vi "Add Item.vi"(0 "Monkeys in":T1, 1 "Item":u64, 2 "Monkey":string) -> (3 "Monkeys out":T1)   [LabVIEW 2020, in "AoC 2022.lvlib"]
uses:
  AoC 2022.lvlib
  Monkeys.ctl
  Monkey.ctl
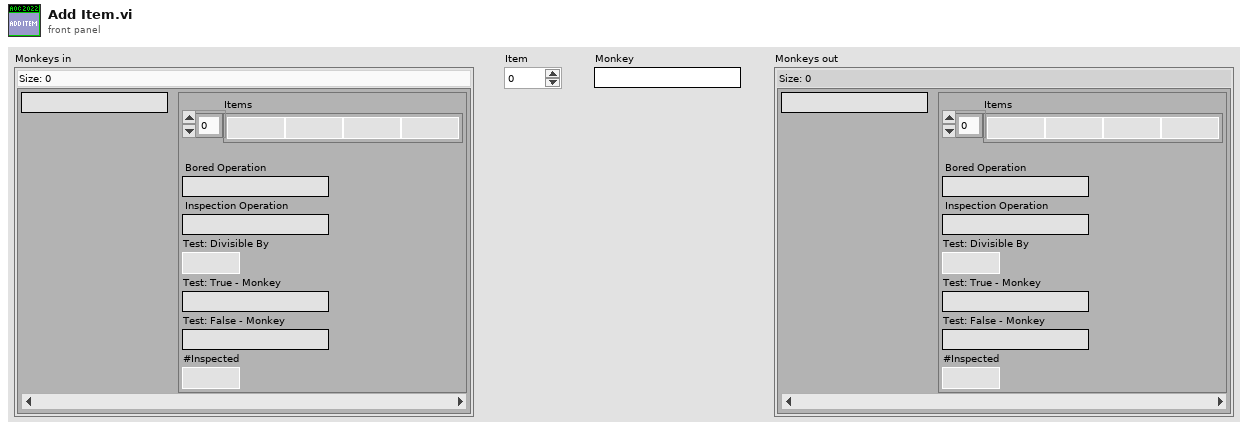
[diagram p1: front panel]
types:
  T1 = typedef "AoC 2022.lvlib/Monkeys.ctl" = map{string, T2}
  T2 = typedef "AoC 2022.lvlib/Monkey.ctl" = cluster{"Items":u64[], "Bored Operation":string, "Inspection Operation":string, "Test: Divisible By":u64, "Test: True - Monkey":string, "Test: False - Monkey":string, "#Inspected":i32}
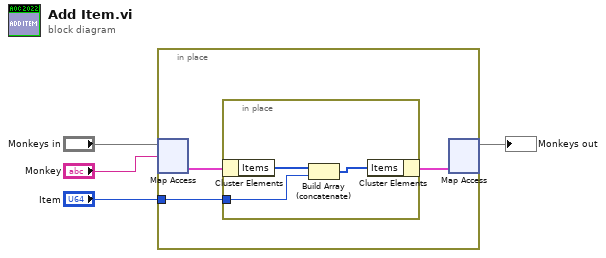
[diagram p0: block diagram]
diagram:
  n1 = in-place {
    in-place-border: "Item" -> [w5]
    n2 = in-place-map #1("Monkeys in", "Monkey") -> (w7:T2)  [unwired: 1 in, 1 out]
    n3 = in-place {
      in-place-border: w5 -> [w8]
      n4 = in-place-cluster #2(w7) -> ("Items"=w10:u64[])
      n5 = Build Array (concatenate)(w10, w8) -> (w9:u64[])
      n6 = in-place-cluster #2("Items"=w9) -> (w6:T2)
    }
    n7 = in-place-map #1(w6) -> (→"Monkeys out":T1)  [unwired: 1 in, 2 out]
  }
